vi "VS_CloseProject.vi"(0 "Engine Reference(in)":refnum<k7>, 1 "Condition Run?":bool, 5 "Sequence File Ref(in)":refnum<k7>, 7 "VeriStand version info":T1, 11 "error in":errorcluster, 12 "Step Group":i32(ring) items=["StepGroup_Setup", "StepGroup_Main", "StepGroup_Cleanup"], 13 "Step Index":i32) -> (4 "Engine reference(out)":refnum<k7>, 6 "Sequence File Ref(out)":refnum<k7>, 8 "VeriStand version info (out)":T1, 15 "error out":errorcluster)   [LabVIEW 2010]
doc: "This VI creates the VeriStand object reference step in TestStand to access the dotNet API. This VI needs to be called always at the beginning of any VeriStand sequence in TestStand"
uses:
  Ctls/dotNetAssemblyInfo.ctl
  Ctls/VSModuleTokens.ctl
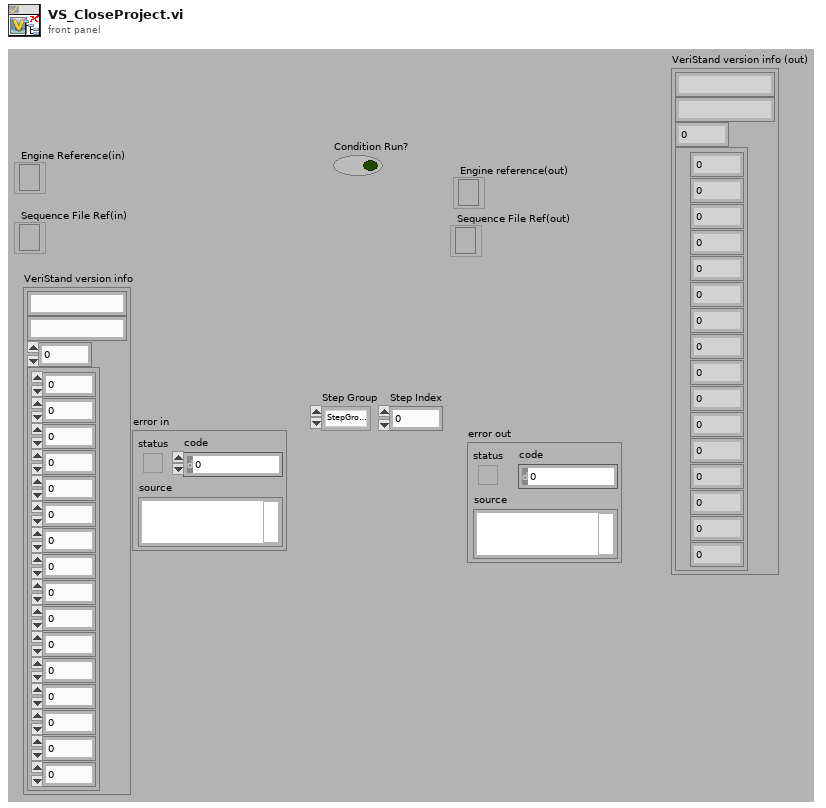
[diagram p1: front panel]
types:
  T1 = typedef "dotNetAssemblyInfo.ctl" = cluster{"VeriStand.exe Path":string, "Assembly":string, "Constructor Token":i32, "Module Token":T2}
  T2 = typedef "VSModuleTokens.ctl" = cluster{"GetIWorkspaceToken":i32, "GetIStimulusToken":i32, "GetIModelManagerToken":i32, "GetIProjectToken":i32, "RunProjectToken":i32, "CloseProjectToken":i32, "RunWorkspaceToken":i32, "StopWorkspaceToken":i32, "SetSingleChannelToken":i32, "SetMultipleParametersToken":i32, "RunStimulusToken":i32, "GetStimulusStateToken":i32, "Open WorkspaceToken":i32, "DeployToken":i32, "UndeployToken":i32, "QuitToken":i32}
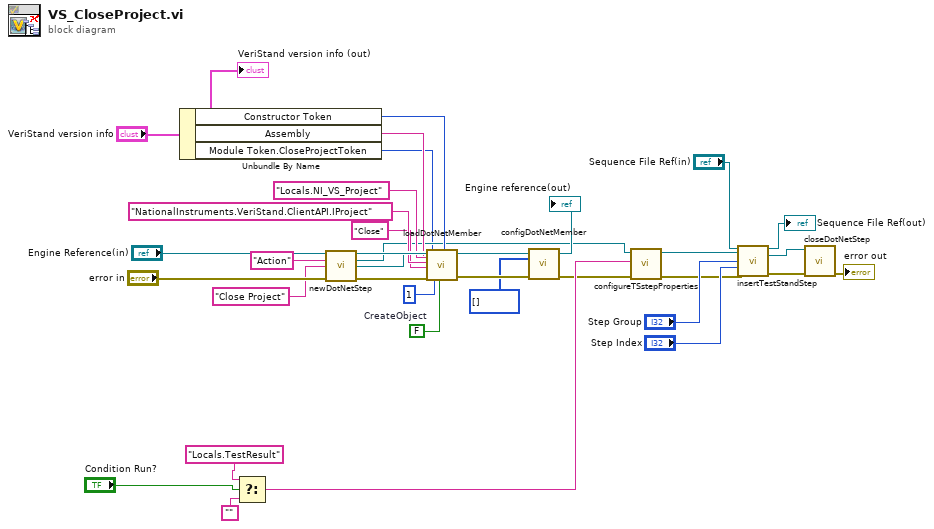
[diagram p0: block diagram]
diagram:
  w18 = FALSE  # CreateObject
  n1 = Unbundle By Name("VeriStand version info") -> ("Constructor Token"=w12:i32, "Assembly"=w13:string, "Module Token.CloseProjectToken"=w1:i32)
  n2 = Select(t="Locals.TestResult", s="Condition Run?", f="") -> (s? t:f=w4:string)
  n3 = call "newDotNetStep.vi"("Engine reference"="Engine Reference(in)", "stepType"="Action", "Step Name"="Close Project", "error in"="error in") -> ("Engine reference(out)"=→"Engine reference(out)":refnum<k7>, "NewStep (out)"=w6:refnum<k7>, "dotNetModule(out)"=w22:refnum<k7>, "error out"=w34:errorcluster)  [unwired: 8 in]
  n4 = call "loadDotNetMember.vi"("dotNetModule"=w22, "Strong Assembly path"=w13, "ClassName"="NationalInstruments.VeriStand.ClientAPI.IProject", "MemberName"="Close", "Member token"=w1, "error in(no error)"=w34, "ClassReference"="Locals.NI_VS_Project", "Call Member?"=1 ("Call Memeber?"), "CreateObject"=w18, "Constructor Token"=w12) -> ("dotNetModule(out)"=w17:refnum<k7>, "error out"=w16:errorcluster)  [unwired: 8 in]
  n5 = call "configDotNetMember.vi"("dotNetModule"=w17, "Index array"=i32[] [], "error in (no error)"=w16) -> ("error out"=w3:errorcluster)  [unwired: 12 in]
  n6 = call "configureTSstepProperties.vi"("error in"=w3, "Precondition"=w4, "NewStep (in)"=w6) -> ("error out"=w2:errorcluster, "NewStep (out)"=w5:refnum<k7>)  [unwired: 7 in]
  n7 = call "insertTestStandStep.vi"("Sequence File Ref"="Sequence File Ref(in)", "Step to insert"=w5, "Step Group"="Step Group", "index"="Step Index", "error out"=w2) -> ("Sequence File Ref(out)"=→"Sequence File Ref(out)":refnum<k7>, "Step to insert (out)"=w33:refnum<k7>, "error out"=w31:errorcluster)  [unwired: 8 in]
  n8 = call "closeDotNetStep.vi"("error in"=w31, "NewStep"=w33) -> ("error out"=→"error out":errorcluster)  [unwired: 9 in]
  "VeriStand version info (out)" <- "VeriStand version info"
